vi "Smooth Spectrum.vi"(11 "FFT In":cluster{"f0":dbl, "df":dbl, "magnitude":dbl[]}[](array[cluster])) -> ()   [LabVIEW 2014]
uses:
  <vilib>/Analysis/NI_AALBase.lvlib
panel:
  in  "Close Button":bool
  out "Waveform Graph 2":dbl[][](graph)
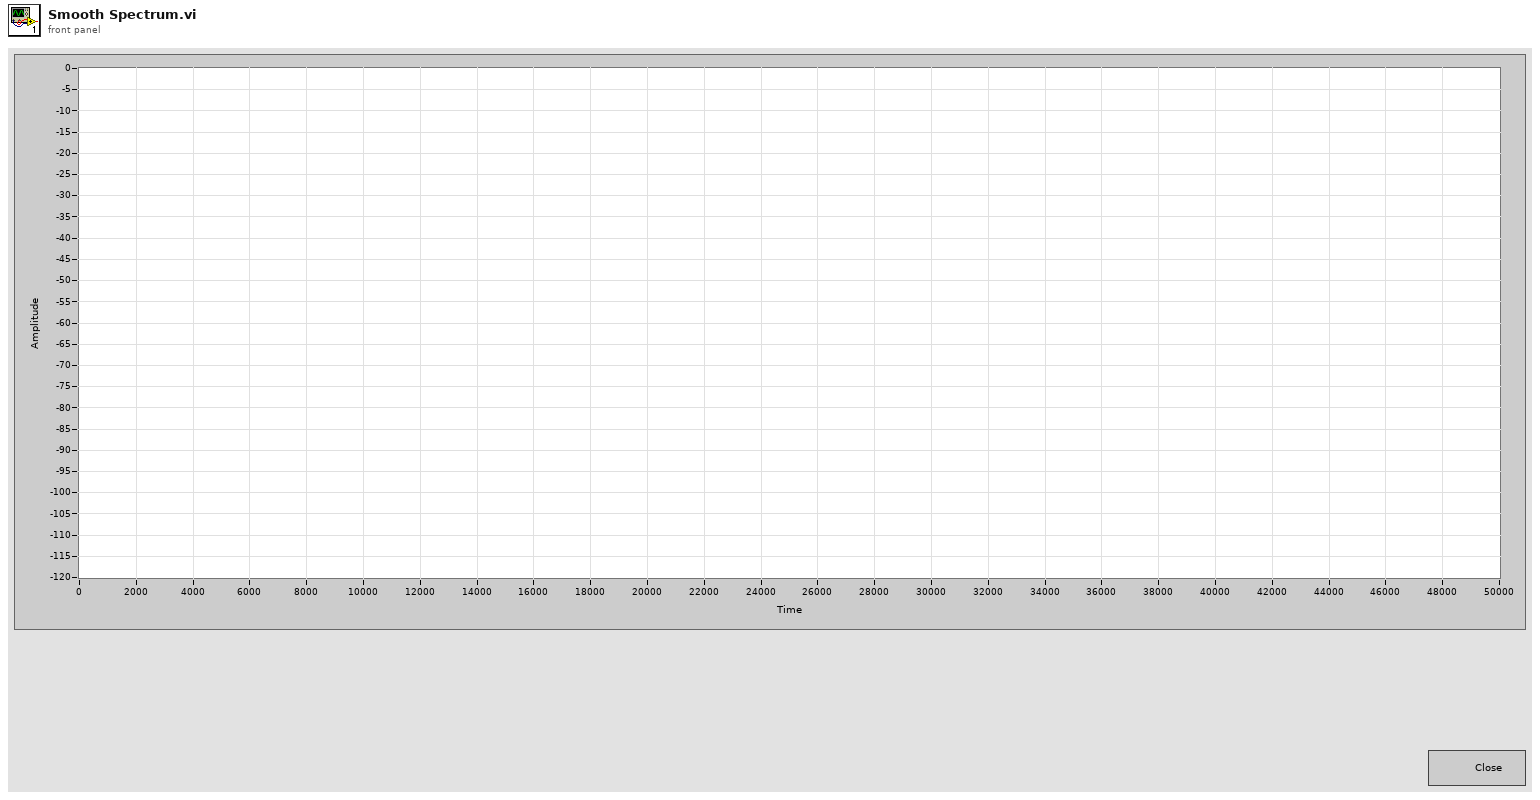
[diagram p1: front panel]
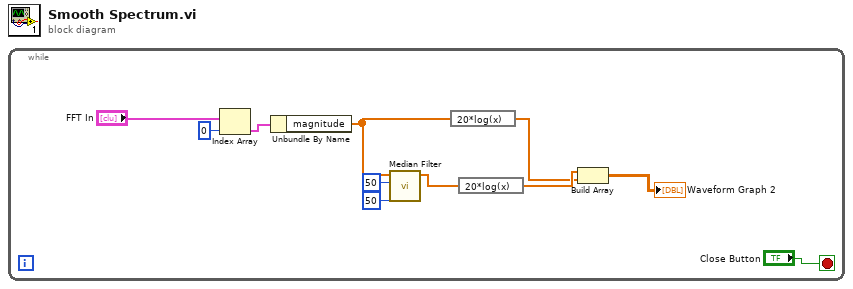
[diagram p0: block diagram]
diagram:
  n1 = while {
    stop <- "Close Button" stop-if-true
    n2 = Index Array(array="FFT In", index=0) -> (element=w11:cluster{"f0":dbl, "df":dbl, "magnitude":dbl[]})
    n3 = Unbundle By Name(w11) -> ("magnitude"=w5:dbl[])
    n4 = call <vilib>:"Median Filter.vi"("right rank"=50, "left rank"=50, "X"=w5) -> ("Filtered X"=w6:dbl[])  [unwired: 7 in, 1 out]
    n5 = expression code="20*log(x)"(w5) -> (w3:dbl[])
    n6 = expression code="20*log(x)"(w6) -> (w4:dbl[])
    n7 = Build Array(w4, w3) -> (→"Waveform Graph 2":dbl[][])
  }
